vi "z to index.vi"(7 "number of points":i32, 10 "complex region":T1, 11 "z":cdb) -> (2 "im index":i32, 3 "re index":i32)   [LabVIEW 2010]
uses:
  complex region.ctl
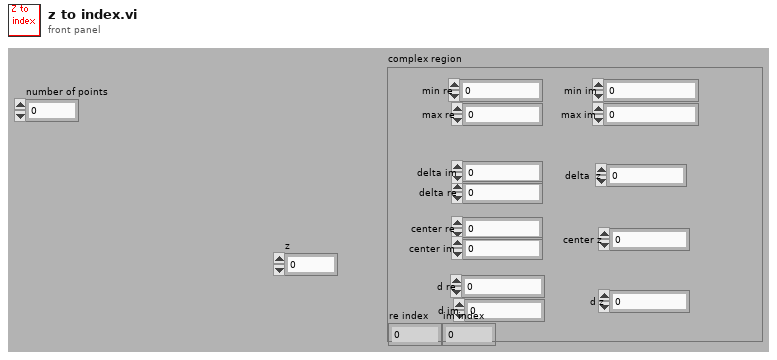
[diagram p1: front panel]
types:
  T1 = typedef "complex region.ctl" = cluster{"max re":dbl, "min re":dbl, "max im":dbl, "min im":dbl, "delta re":dbl, "delta im":dbl, "center re":dbl, "delta  z":cdb, "center im":dbl, "center z":cdb, "d im":dbl, "d re":dbl, "d z":cdb}
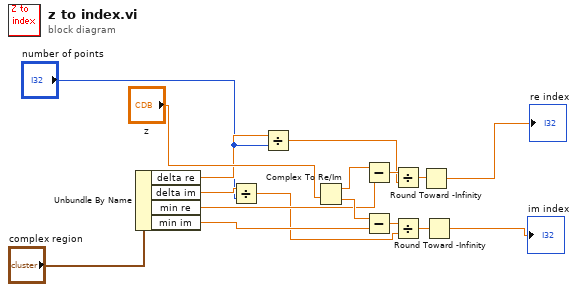
[diagram p0: block diagram]
diagram:
  n1 = Unbundle By Name("complex region") -> ("delta re"=w5:dbl, "delta im"=w3:dbl, "min re"=w11:dbl, "min im"=w10:dbl)
  n2 = Divide(x=w3, y="number of points") -> (x/y=w1:dbl)
  n3 = Divide(x=w5, y="number of points") -> (x/y=w4:dbl)
  n4 = Complex To Re/Im(x + iy="z") -> (x=w17:dbl, y=w14:dbl)
  n5 = Subtract(x=w17, y=w11) -> (x-y=w16:dbl)
  n6 = Subtract(x=w14, y=w10) -> (x-y=w15:dbl)
  n7 = Divide(x=w16, y=w4) -> (x/y=w13:dbl)
  n8 = Divide(x=w15, y=w1) -> (x/y=w12:dbl)
  n9 = Round Toward -Infinity(1:w13) -> (0:→"re index":dbl)
  n10 = Round Toward -Infinity(1:w12) -> (0:→"im index":dbl)
